vi "Keys to pattern list.vi"(10 "Keys":string[](array[string])) -> (2 "Pattern List":string[](array[string]))   [LabVIEW 2018, in "Configuration.lvlib"]
uses:
  Configuration.lvlib
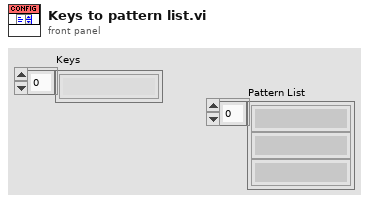
[diagram p1: front panel]
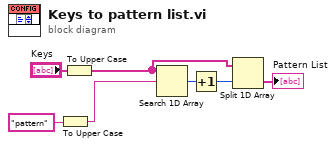
[diagram p0: block diagram]
diagram:
  n1 = To Upper Case(1:"pattern" ("element")) -> (0:w5:string)
  n2 = To Upper Case(1:"Keys") -> (0:w4:string[])
  n3 = Search 1D Array(1D array=w4, element=w5) -> (index of element=w3:i32)  [unwired: 1 in]
  n4 = Increment(x=w3) -> (x+1=w1:i32)
  n5 = Split 1D Array(array=w4, index=w1) -> (second subarray=→"Pattern List":string[])  [unwired: 1 out]
